vi "Pack For Grpc.vi"(8 "error in (no error)":errorcluster, 9 "Configuration / Resuls (Config)":enum16{"Configuration", "Results"}(ring), 10 "Data Value":variant, 11 "Measurement Customizations in":refnum<class "MeasurementPlugin.lvclass">) -> (0 "error out":errorcluster, 2 "Any":T1, 3 "Measurement Customizations out":refnum<class "MeasurementPlugin.lvclass">)   [LabVIEW 2021, in "audio_adc_acMeasurement.lvlib" / "MeasurementPlugin.lvclass"]
uses:
  MeasurementPlugin.lvclass
  <vilib>/gRPC/LabVIEW gRPC Library/Shared/Any.ctl
  Measurement Configuration.ctl
  Measurement Results.ctl
  2eca732d-dbaa-43bf-a7dd-ede2da65bc1b.vi
  a6012965-5700-4384-8228-972e71b6560c.vi
  <vilib>/gRPC/LabVIEW gRPC Library/Server API/Translate Protobuf Error.vi
  <vilib>/AdvancedString/1D String Array to Delimited String.vi
  <vilib>/gRPC/LabVIEW gRPC Library/Server API/Server/Get Server DLL Path.vi
  audio_adc_acMeasurement.lvlib
  <vilib>/gRPC/LabVIEW gRPC Library/grpc-lvsupport-release.lvlib
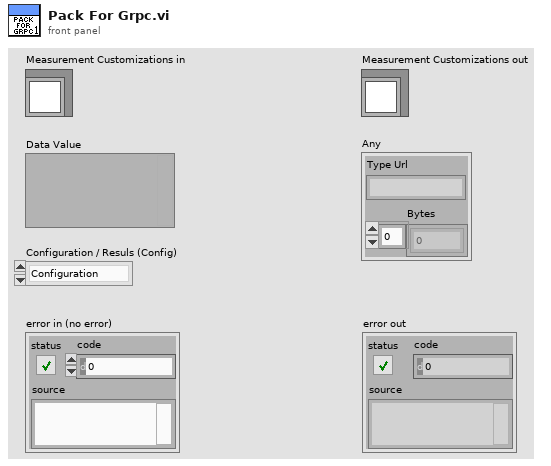
[diagram p1: front panel]
types:
  T1 = typedef "grpc-lvsupport-release.lvlib/Any.ctl" = cluster{"Type Url":string, "Bytes":u8[]}
  T2 = typedef "grpc-lvsupport-release.lvlib/grpcId.ctl" = u64
  T3 = typedef "audio_adc_acMeasurement.lvlib/Measurement Configuration.ctl" = cluster{"Band start":dbl, "Band stop":dbl, "Weighting filter":string, "Amplitude":dbl, "Frequency":dbl, "Full scale range":dbl, "Analog source resource name":string, "Protocol capture resource name":string, "Channel name":string, "Data line":u16, "Sample rate":dbl, "Measurement duration":dbl, "Channel":u32, "Frame sync edge for channel 0":u32, "Channel count per frame":u32, "Channel length":u32, "Bit depth":u32, "Channel 0 offset":u32, "Endianness":u32, "Data justification":u32, "Frame length":u32, "Frame sync pulse width":u32, "Bit clock edge sync":u32}
  T4 = typedef "audio_adc_acMeasurement.lvlib/Measurement Results.ctl" = cluster{"Channel":string, "Calculated frequency":dbl, "Calculated amplitude":dbl, "SNR":dbl, "THD+N":dbl, "THD":dbl, "Dynamic range":dbl, "Gain error":dbl, "SFDR":dbl, "t0":dbl, "dt":dbl, "Time domain":dbl[], "f0":dbl, "df":dbl, "Spectrum":dbl[]}
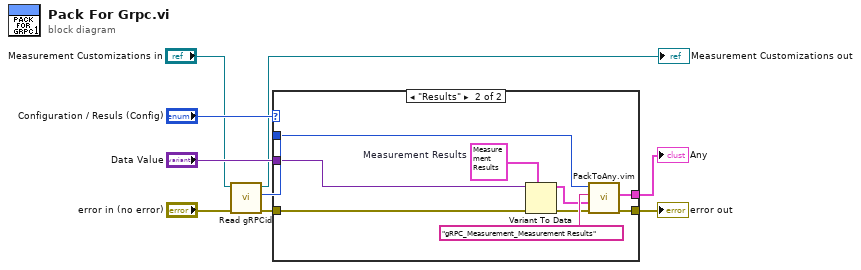
[diagram p0: block diagram]
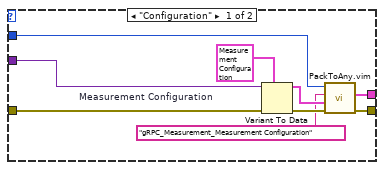
[diagram p2: hidden frame]
diagram:
  n1 = call-dynamic "Read gRPCid.vi"("error in (no error)"="error in (no error)", "MeasurementPluginService in"="Measurement Customizations in") -> ("error out"=w4:errorcluster, "gRPCid"=w1:T2, "MeasurementPluginService out"=→"Measurement Customizations out":refnum<class "MeasurementPlugin.lvclass">)  [unwired: 7 in]
  n2 = case shown="\"Results\"" "Configuration / Resuls (Config)" {
    tunnel: w4 -> [w18 w27]
    tunnel: "Data Value" -> [w17 w26]
    tunnel: w1 -> [w14 w22]
    tunnel: [w16 w24] -> w8
    tunnel: [w15 w23] -> w7
    frame "Configuration" {
      w11 = T3 {"Band start"=20.0, "Band stop"=20000.0, "Weighting filter"="", "Amplitude"=1.0, "Frequency"=1000.0, "Full scale range"=3.16, "Analog source resource name"="", "Protocol capture resource name"="PXI1Slot7\\I2Si 0", "Channel name"="", "Data line"=0, "Sample rate"=12288000.0, "Measurement duration"=19200.0, "Channel"=0, "Frame sync edge for channel 0"=1, "Channel count per frame"=2, "Channel length"=32, "Bit depth"=24, "Channel 0 offset"=1, "Endianness"=0, "Data justification"=0, "Frame length"=64, "Frame sync pulse width"=32, "Bit clock edge sync"=1}  # Measurement Configuration
      n3 = Variant To Data(error in=w18, type=w11, Variant=w17) -> (data=w13:T3, error out=w12:errorcluster)
      n4 = call "PackToAny.vim"("error in"=w12, "Data To Pack"=w13, "Message Type"="gRPC_Measurement_Measurement Configuration", "gRPCid in"=w14) -> ("error out"=w16:errorcluster, "Any"=w15:T1)  [unwired: 5 in, 1 out]
    }
    frame "Results" {
      w25 = T4 {"Channel"="", "Calculated frequency"=0.0, "Calculated amplitude"=0.0, "SNR"=0.0, "THD+N"=0.0, "THD"=0.0, "Dynamic range"=0.0, "Gain error"=0.0, "SFDR"=0.0, "t0"=0.0, "dt"=0.0, "Time domain"=[], "f0"=0.0, "df"=0.0, "Spectrum"=[]}  # Measurement Results
      n5 = Variant To Data(error in=w27, type=w25, Variant=w26) -> (data=w20:T4, error out=w19:errorcluster)
      n6 = call "PackToAny.vim"("error in"=w19, "Data To Pack"=w20, "Message Type"="gRPC_Measurement_Measurement Results", "gRPCid in"=w22) -> ("error out"=w24:errorcluster, "Any"=w23:T1)  [unwired: 5 in, 1 out]
    }
  }
  "error out" <- w8
  "Any" <- w7
